vi "工位2扫码.vi"(7 "工位1逻辑与":bool, 9 "工位1表格":string[][](array[string]), 10 "46~99编号数组":string[](array[string]), 11 "MulticolumnListbox输入":refnum<vi>) -> (1 "有空料？":bool, 2 "条码字符串":string, 3 "工位2NG?":bool, 5 "1~99保存报表":string[][](array[string]))   [LabVIEW 2014]
uses:
  <vilib>/Utility/miscctls.llb/LVRowAndColumnTypeDef.ctl
panel:
  out "已删除的部分 2":string[](array[string])
  out "已删除元素的数组子集 2":string[](array[string])
  out "元素索引 2":i32
  out "工位1逻辑与 2":bool
  out "料号":string[](array[string])
  out "1~45编号数组":string[](array[string])
  out "?":string[][](array[string])
  out "转置的数组":string[][](array[string])
  in  "多列列表框 2":i32[](listbox)
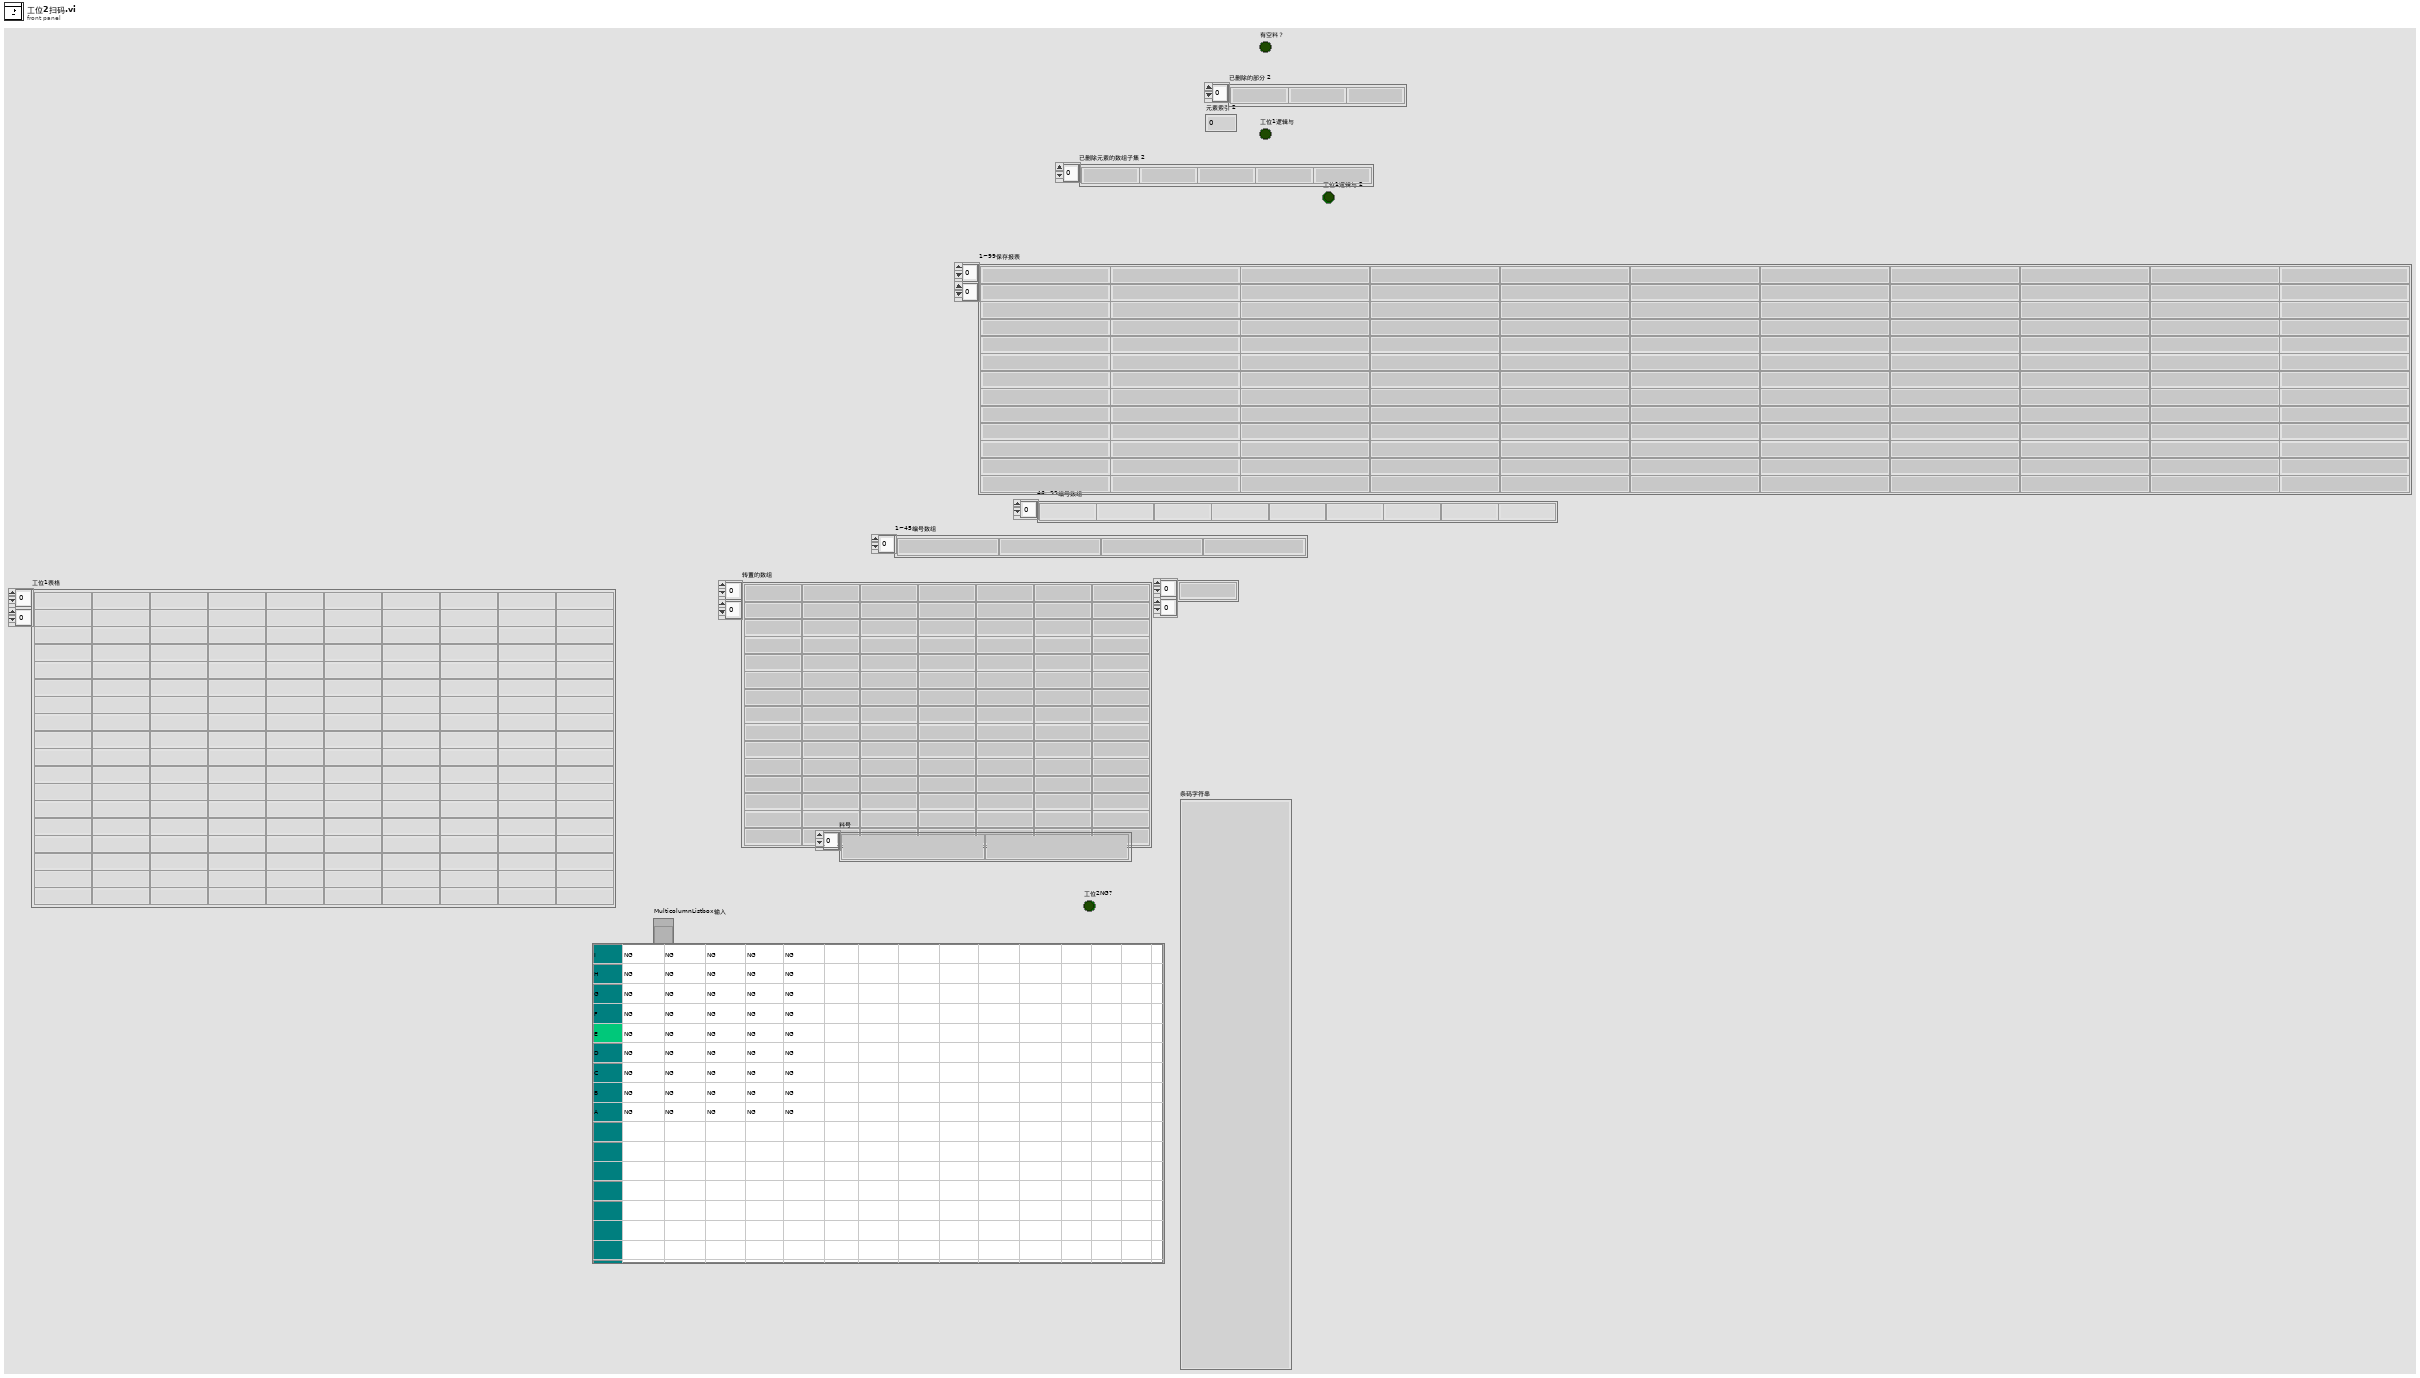
[diagram p1: front panel]
types:
  T1 = typedef "LVRowAndColumnTypeDef.ctl" = cluster{"Row":i32, "Column":i32}
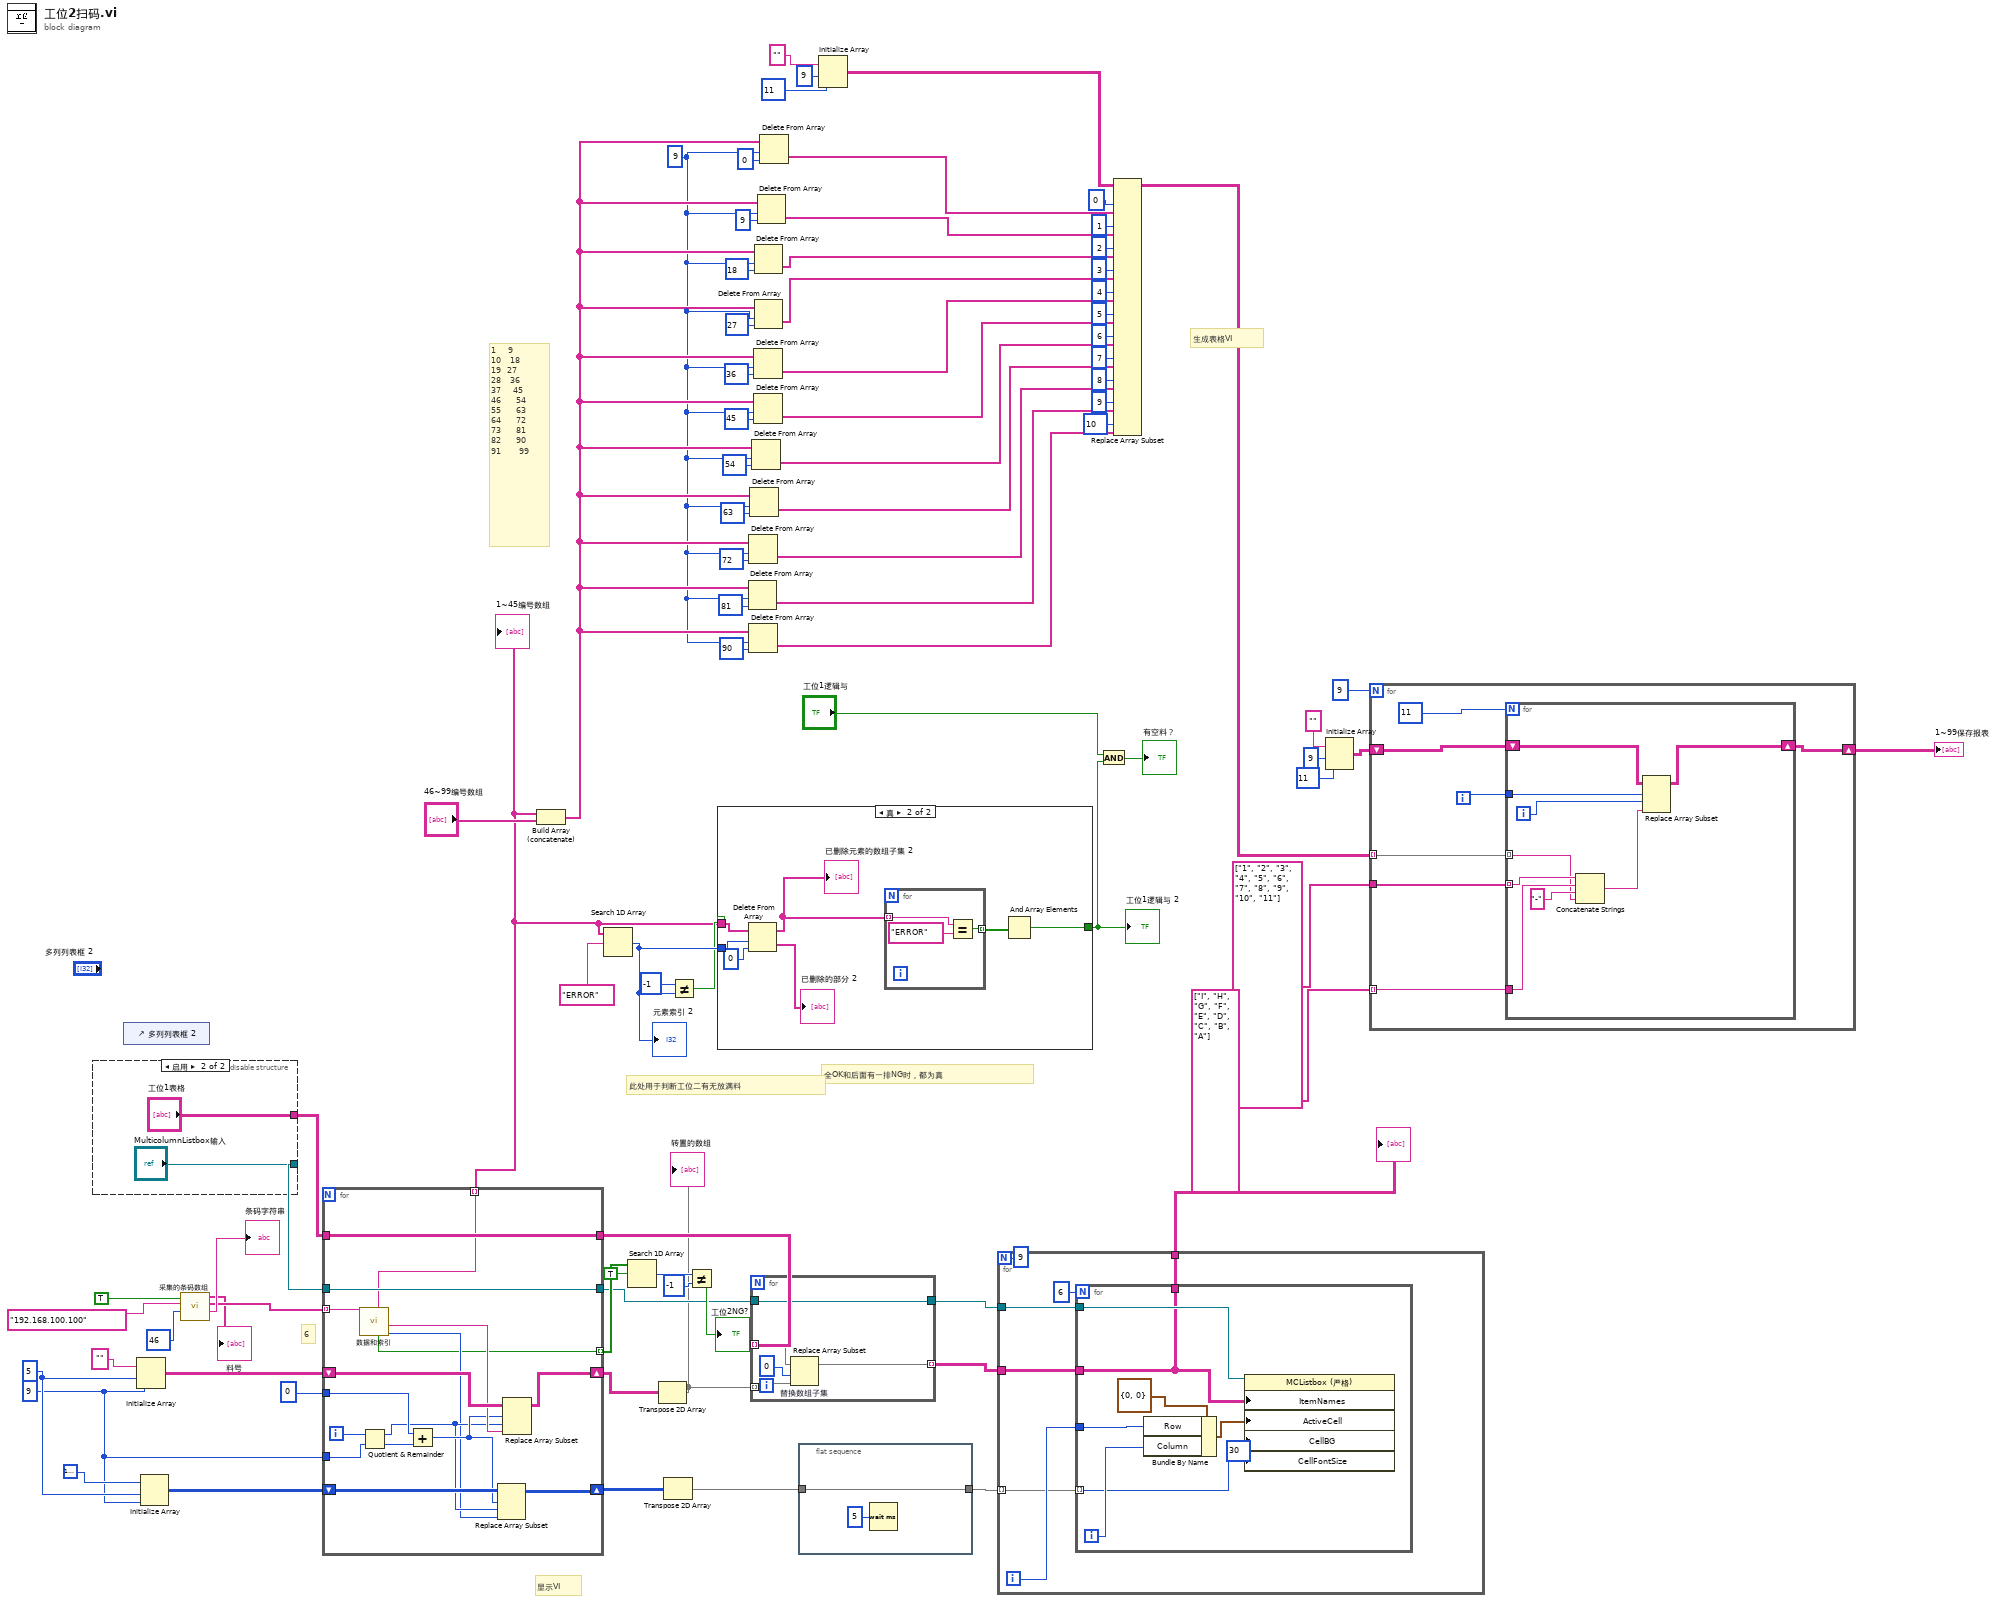
[diagram p0: block diagram]
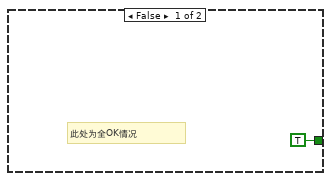
[diagram p2: hidden frame]
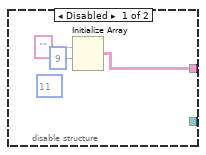
[diagram p3: hidden frame]
diagram:
  w52 = 9 ("长度")
  w78 = 9 ("维数大小")
  w79 = 5 ("维数大小")
  # "全OK和后面有一排NG时，都为真"
  # "显示VI"
  # "生成表格VI"
  # "此处用于判断工位二有无放满料"
  # "1    9\n10   18\n19  27\n28   36\n37    45\n46     54\n55     63\n64     72\n73     81\n82     90\n91      99"
  # "6"
  n1 = disable-structure shown="启用" {
    disable-tunnel: [w90 "工位1表格"] -> w59
    disable-tunnel: [w89 "MulticolumnListbox输入"] -> w60
    frame Disabled {
      (unwired) 11 ("维数大小")
      n2 = Initialize Array("", 9 ("维数大小")) -> (w90:string[][])  [unwired: 1 in]
    }
    frame Enabled {
    }
  }
  n3 = control-ref of="多列列表框 2"() -> ()  [unwired: 1 out]
  n4 = Initialize Array("", w79, w78) -> (w83:string[][])
  n5 = Initialize Array(u32 16777238, w79, w78) -> (w81:u32[][])
  n6 = call "采集的条码数组.vi"("条码数量"=46, "地址"="192.168.100.100", "开启条码?"=TRUE) -> ("条码字符串"=→"条码字符串":string, "条码数组"=w85:string[], "料号"=→"料号":string[])  [unwired: 6 in]
  n7 = for {
    tunnel: w85 -> [w106] mode=indexing
    shift-right: [w99] -> w77
    shift-left: w83 -> [w107]
    shift-right: [w98] -> w76
    shift-left: w81 -> [w104]
    tunnel: 0 -> [w108]
    tunnel: w78 -> [w110]
    tunnel: [w100] -> w72 mode=indexing
    tunnel: w60 -> [w97]
    tunnel: [w97] -> w67
    tunnel: w59 -> [w96]
    tunnel: [w96] -> w71
    tunnel: [w95] -> w4 mode=indexing
    i -> [w111]
    n8 = call "数据和索引.vi"("data out"=w106) -> ("颜色"=w101:u32, "显示数据"=w105:string, "NG?"=w100:bool, "条码"=w95:string)  [unwired: 6 in, 1 out]
    n9 = Quotient & Remainder(x=w111, y=w110) -> (x-y*floor(x/y)=w102:i32, floor(x/y)=w109:i32)
    n10 = Add(x=w108, y=w109) -> (x+y=w103:i32)
    n11 = Replace Array Subset(array=w104, new element=w101, index (row)=w103, index (col)=w102) -> (w98:u32[][])
    n12 = Replace Array Subset(array=w107, new element=w105, index (row)=w103, index (col)=w102) -> (w99:string[][])
  }
  "1~45编号数组" <- w4
  n13 = Build Array (concatenate)(w4, "46~99编号数组") -> (w53:string[])
  n14 = Search 1D Array(1D array=w4, element="ERROR") -> (index of element=w7:i32)  [unwired: 1 in]
  "元素索引 2" <- w7
  n15 = Search 1D Array(1D array=w72, element=TRUE) -> (index of element=w74:i32)  [unwired: 1 in]
  n16 = Transpose 2D Array(2D array=w77) -> (transposed array=w62:string[][])
  "转置的数组" <- w62
  n17 = Transpose 2D Array(2D array=w76) -> (transposed array=w70:u32[][])
  n18 = Not Equal?(x=-1, y=w7) -> (x != y?=w6:bool)
  n19 = Not Equal?(x=w74, y=-1) -> (x != y?=→"工位2NG?":bool)
  n20 = case shown="真" w6 {
    tunnel: [TRUE w119] -> w3
    tunnel: w4 -> [_ w118]
    tunnel: w7 -> [_ w117]
    frame False {
      # "此处为全OK情况"
    }
    frame True {
      n21 = Delete From Array(array=w118, length=w117, index=0 ("索引")) -> (deleted portion=→"已删除的部分 2":string[], array with subset deleted=w114:string[])
      "已删除元素的数组子集 2" <- w114
      n22 = for {
        tunnel: w114 -> [w122] mode=indexing
        tunnel: [w120] -> w113 mode=indexing
        n23 = Equal?(x=w122, y="ERROR") -> (x = y?=w120:bool)
      }
      n24 = And Array Elements(Boolean array=w113) -> (logical AND=w119:bool)
    }
  }
  "工位1逻辑与 2" <- w3
  n25 = Delete From Array(array=w53, length=w52, index=81 ("索引")) -> (deleted portion=w27:string[])  [unwired: 1 out]
  n26 = Delete From Array(array=w53, length=w52, index=72 ("索引")) -> (deleted portion=w28:string[])  [unwired: 1 out]
  n27 = Delete From Array(array=w53, length=w52, index=90 ("索引")) -> (deleted portion=w26:string[])  [unwired: 1 out]
  n28 = Delete From Array(array=w53, length=w52, index=63 ("索引")) -> (deleted portion=w29:string[])  [unwired: 1 out]
  n29 = for {
    tunnel: w62 -> [w126] mode=indexing
    tunnel: w71 -> [w127] mode=indexing
    tunnel: [w124] -> w68 mode=indexing
    tunnel: w67 -> [w123]
    tunnel: [w123] -> w66
    n30 = Replace Array Subset "替换数组子集"(array=w127, new element=w126, index=0 ("索引")) -> (w124:string[])
  }
  n31 = Delete From Array(array=w53, length=w52, index=54 ("索引")) -> (deleted portion=w30:string[])  [unwired: 1 out]
  n32 = Delete From Array(array=w53, length=w52, index=36 ("索引")) -> (deleted portion=w32:string[])  [unwired: 1 out]
  n33 = Delete From Array(array=w53, length=w52, index=45 ("索引")) -> (deleted portion=w31:string[])  [unwired: 1 out]
  n34 = Delete From Array(array=w53, length=w52, index=18 ("索引")) -> (deleted portion=w35:string[])  [unwired: 1 out]
  n35 = Delete From Array(array=w53, length=w52, index=27 ("索引")) -> (deleted portion=w33:string[])  [unwired: 1 out]
  n36 = Delete From Array(array=w53, length=w52, index=9 ("索引")) -> (deleted portion=w34:string[])  [unwired: 1 out]
  n37 = Delete From Array(array=w53, length=w52, index=0 ("索引")) -> (deleted portion=w37:string[])  [unwired: 1 out]
  n38 = flat-sequence {
    tunnel: w70 -> [w129]
    tunnel: [w129] -> w65
    frame #0 {
      n39 = Wait (ms)(milliseconds to wait=u32 5 ("等待时间（毫秒）")) -> ()  [unwired: 1 out]
    }
  }
  n40 = Initialize Array("", 9 ("维数大小"), 11 ("维数大小")) -> (w38:string[][])
  n41 = for {
    N: 9 -> [_]
    tunnel: w68 -> [w134]
    tunnel: w66 -> [w135]
    tunnel: w65 -> [w131] mode=indexing
    tunnel: [w130] -> w61
    i -> [w132]
    n42 = for {
      N: 6 -> [_]
      tunnel: w135 -> [w143]
      tunnel: w134 -> [w136]
      tunnel: w132 -> [w140]
      tunnel: w131 -> [w138] mode=indexing
      tunnel: [w136] -> w130
      i -> [w139]
      n43 = Bundle By Name(cluster=T1 {"Row"=0, "Column"=0} ("活动单元格:活动单元格"), "Row"=w140, "Column"=w139) -> (w141:T1)
      n44 = property class="MCListbox (严格)"(reference=w143, "ItemNames"=w136, "ActiveCell"=w141, "CellBG"=w138, "CellFontSize"=u32 30 ("活动单元格:单元格字体:字号")) -> ()  [unwired: 1 in, 2 out]
    }
  }
  "?" <- w61
  n45 = And(x="工位1逻辑与", y=w3) -> (x .and. y?=→"有空料？":bool)
  n46 = Replace Array Subset(array=w38, new element #1=w37, index (col) #1=0 ("禁用的索引 (列)"), new element #2=w34, index (col) #2=1 ("索引 (列)"), new element #3=w35, index (col) #3=2 ("索引 (列)"), new element #4=w33, index (col) #4=3 ("索引 (列)"), new element #5=w32, index (col) #5=4 ("索引 (列)"), new element #6=w31, index (col) #6=5 ("索引 (列)"), new element #7=w30, index (col) #7=6 ("索引 (列)"), new element #8=w29, index (col) #8=7 ("索引 (列)"), new element #9=w28, index (col) #9=8 ("索引 (列)"), new element #10=w27, index (col) #10=9 ("索引 (列)"), new element #11=w26, index (col) #11=10 ("索引 (列)")) -> (w15:string[][])  [unwired: 11 in]
  n47 = Initialize Array("", 9 ("维数大小"), 11 ("维数大小")) -> (w11:string[][])
  n48 = for {
    N: 9 -> [_]
    tunnel: w15 -> [w149] mode=indexing
    tunnel: string[] ["1", "2", "3", "4", "5", "6", "7", "8", "9", "10", "11"] -> [w146]
    tunnel: string[] ["I", "H", "G", "F", "E", "D", "C", "B", "A"] -> [w145] mode=indexing
    shift-right: [w144] -> w10
    shift-left: w11 -> [w150]
    i -> [w148]
    n49 = for {
      N: 11 -> [_]
      tunnel: w149 -> [w153] mode=indexing
      tunnel: w148 -> [w158]
      tunnel: w146 -> [w156] mode=indexing
      tunnel: w145 -> [w155]
      shift-right: [w151] -> w144
      shift-left: w150 -> [w159]
      i -> [w157]
      n50 = Concatenate Strings(w156, w155, "-", w153) -> (w152:string)
      n51 = Replace Array Subset(array=w159, new element=w152, index (row)=w158, index (col)=w157) -> (w151:string[][])
    }
  }
  "1~99保存报表" <- w10
